vi "Calculator.vi"(1 "Wait (ms)":dbl, 2 "Input 2":dbl, 3 "Input 1":dbl) -> (0 "Decimal Result":dbl)   [LabVIEW 2012]
panel:
  out "Binary Result":i16[](array[numeric])
  out "Result Voltages":dbl[](array[numeric])
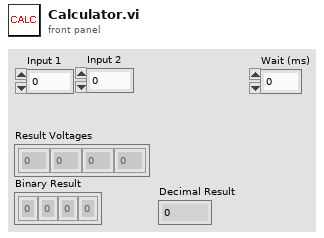
[diagram p1: front panel]
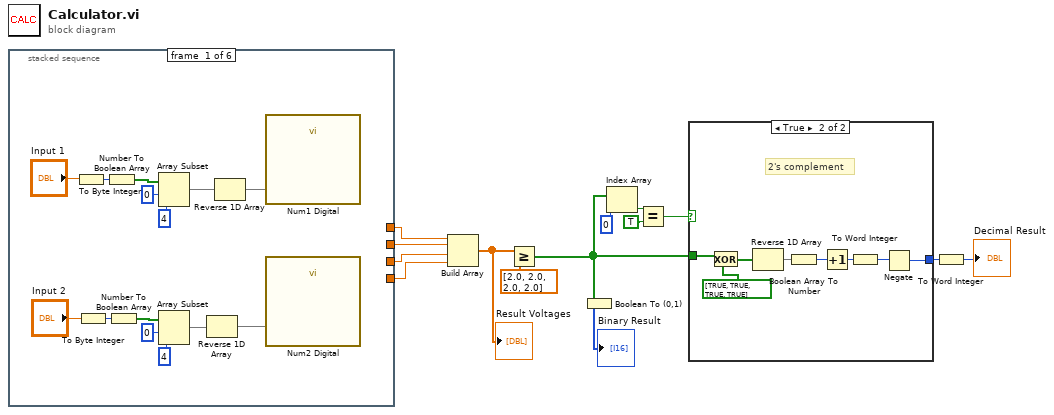
[diagram p0: block diagram]
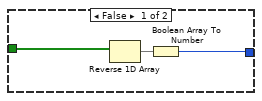
[diagram p2: hidden frame]
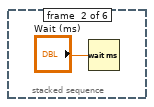
[diagram p3: hidden frame]
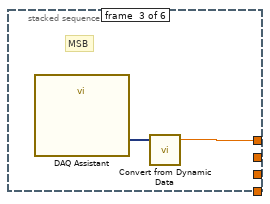
[diagram p4: hidden frame]
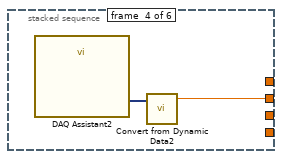
[diagram p5: hidden frame]
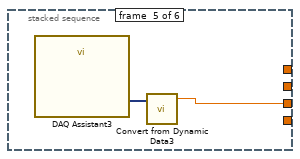
[diagram p6: hidden frame]
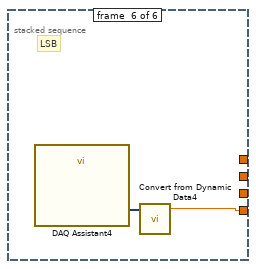
[diagram p7: hidden frame]
diagram:
  n1 = stacked-sequence {
    tunnel: [_ _ w30 _ _ _] -> w14
    tunnel: [_ _ _ w32 _ _] -> w13
    tunnel: [_ _ _ _ w34 _] -> w12
    tunnel: [_ _ _ _ _ w36] -> w11
    frame #0 {
      n2 = To Byte Integer(number="Input 1") -> (8bit integer=w27:i8)
      n3 = To Byte Integer(number="Input 2") -> (8bit integer=w23:i8)
      n4 = Number To Boolean Array(number=w27) -> (Boolean array=w26:bool[])
      n5 = Number To Boolean Array(number=w23) -> (Boolean array=w22:bool[])
      n6 = Array Subset(array=w26, index=0, length=4) -> (w16:bool[])
      n7 = Array Subset(array=w22, index=0, length=4) -> (w18:bool[])
      n8 = Reverse 1D Array(array=w18) -> (reversed array=w17:bool[])
      n9 = Reverse 1D Array(array=w16) -> (reversed array=w15:bool[])
      n10 = call "Num1 Digital"("data"=w15) -> ()  [unwired: 17 in, 2 out]
      n11 = call "Num2 Digital"("data"=w17) -> ()  [unwired: 17 in, 2 out]
    }
    frame #1 {
      n12 = Wait (ms)(milliseconds to wait="Wait (ms)") -> ()  [unwired: 1 out]
    }
    frame #2 {
      # "MSB"
      n13 = call "DAQ Assistant"() -> ("data"=w31:dynamicdata)  [unwired: 17 in, 2 out]
      n14 = call "Convert from Dynamic Data"("Dynamic Data Type"=w31) -> ("Scalar"=w30:dbl)  [unwired: 3 in]
    }
    frame #3 {
      n15 = call "DAQ Assistant2"() -> ("data"=w33:dynamicdata)  [unwired: 17 in, 2 out]
      n16 = call "Convert from Dynamic Data2"("Dynamic Data Type"=w33) -> ("Scalar"=w32:dbl)  [unwired: 3 in]
    }
    frame #4 {
      n17 = call "DAQ Assistant3"() -> ("data"=w35:dynamicdata)  [unwired: 17 in, 2 out]
      n18 = call "Convert from Dynamic Data3"("Dynamic Data Type"=w35) -> ("Scalar"=w34:dbl)  [unwired: 3 in]
    }
    frame #5 {
      # "LSB"
      n19 = call "DAQ Assistant4"() -> ("data"=w37:dynamicdata)  [unwired: 17 in, 2 out]
      n20 = call "Convert from Dynamic Data4"("Dynamic Data Type"=w37) -> ("Scalar"=w36:dbl)  [unwired: 3 in]
    }
  }
  n21 = Build Array(w14, w13, w12, w11) -> (w10:dbl[])
  "Result Voltages" <- w10
  n22 = Greater Or Equal?(x=w10, y=dbl[] [2.0, 2.0, 2.0, 2.0]) -> (x >= y?=w3:bool[])
  n23 = Boolean To (0,1)(Boolean=w3) -> (0, 1=→"Binary Result":i16[])
  n24 = Index Array(array=w3, index=0) -> (element=w5:bool)
  n25 = Equal?(x=w5, y=TRUE) -> (x = y?=w6:bool)
  n26 = case shown="True" w6 {
    tunnel: w3 -> [w39 w48]
    tunnel: [w38 w43] -> w2
    frame False {
      n27 = Reverse 1D Array(array=w39) -> (reversed array=w40:bool[])
      n28 = Boolean Array To Number(Boolean array=w40) -> (number=w38:u32)
    }
    frame True {
      # "2's complement"
      n29 = Exclusive Or(1:bool[] [TRUE, TRUE, TRUE, TRUE] ("y"), 2:w48) -> (0:w46:bool[])
      n30 = Reverse 1D Array(array=w46) -> (reversed array=w47:bool[])
      n31 = Boolean Array To Number(Boolean array=w47) -> (number=w45:u32)
      n32 = Increment(x=w45) -> (x+1=w42:u32)
      n33 = To Word Integer(number=w42) -> (16bit integer=w41:i16)
      n34 = Negate(x=w41) -> (-x=w43:i16)
    }
  }
  n35 = To Word Integer(number=w2) -> (16bit integer=→"Decimal Result":i16)
